vi "CreateAc.vi"(0 "Abrupt Change":refnum<class "AbruptChange.lvclass">, 5 "error in (no error)":errorcluster, 6 "default value":dbl, 8 "size (10)":u32, 10 "AlarmType":T1=enum."Alarm", 12 "Tags":T2, 13 "Logger":refnum<class "Logger.lvclass">) -> (14 "AnalogComparator out":refnum<class "AbruptChange.lvclass">, 19 "error out":errorcluster)   [LabVIEW 2019, in "AbruptChange.lvclass"]
uses:
  AbruptChange.lvclass
  D:/GIT H4000/H4000/src/Signal_class/Signal.lvclass
  Proccess_class/TAGs.ctl
  Logger_class/Logger.lvclass
  TypeDef/AlarmType.ctl
  AbruptChange.lvclass/AbruptChange.ctl
  Signal_class/Signal.lvclass
  Proccess_class/Proccess.lvclass
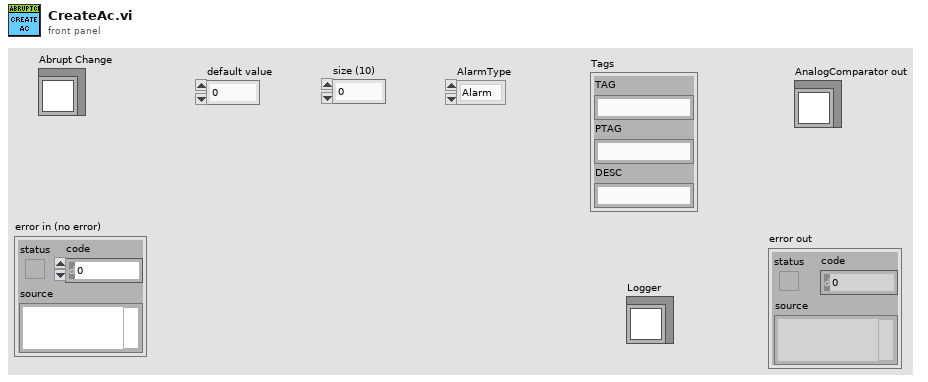
[diagram p1: front panel]
types:
  T1 = typedef "AlarmType.ctl" = enum16{"Normal", "Warning", "Alarm"}
  T2 = typedef "Proccess.lvclass/TAGs.ctl" = cluster{"TAG":string, "PTAG":string, "DESC":string}
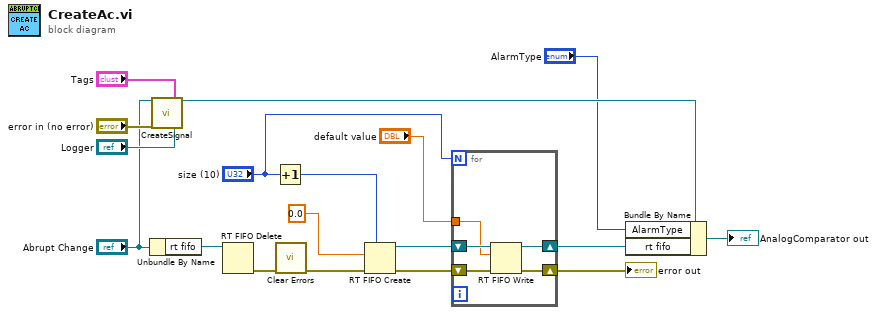
[diagram p0: block diagram]
diagram:
  n1 = Unbundle By Name("Abrupt Change") -> ("rt fifo"=w9:refnum<k33>)
  n2 = call "CreateSignal.vi"("Signal in"="Abrupt Change", "error in (no error)"="error in (no error)", "Tags"="Tags", "Logger"="Logger") -> ("Signal out"=w15:refnum<class "AbruptChange.lvclass">)  [unwired: 14 in, 1 out]
  n3 = RT FIFO Delete(0:w9) -> (11:w11:errorcluster)  [unwired: 2 in]
  n4 = Increment(x="size (10)") -> (x+1=w7:u32)
  n5 = call <vilib>:"Clear Errors.vi"("error in (no error)"=w11) -> ("error out"=w8:errorcluster)  [unwired: 5 in, 1 out]
  n6 = RT FIFO Create(1:0.0, 3:w8, 4:w7) -> (8:w6:refnum<k33>, 11:w5:errorcluster)  [unwired: 5 in, 1 out]
  n7 = for {
    N: "size (10)" -> [_]
    shift-right: [w22] -> w1
    shift-left: w6 -> [w23]
    shift-right: [w20] -> w4
    shift-left: w5 -> [w21]
    tunnel: "default value" -> [w19]
    n8 = RT FIFO Write(0:w23, 1:w19, 3:w21) -> (8:w22:refnum<k33>, 11:w20:errorcluster)  [unwired: 2 in, 2 out]
  }
  "error out" <- w4
  n9 = Bundle By Name(cluster=w15, "AlarmType"="AlarmType", "rt fifo"=w1) -> (→"AnalogComparator out":refnum<class "AbruptChange.lvclass">)
